vi "RT Main R4.vi"() -> ()   [LabVIEW 2018]
uses:
  Type Defs/Measurement States.ctl
  Type Defs/Control Mode.ctl
  <vilib>/FPGAPlugInAG/myRIO-1900/niLvFpga_Open_myRIO-1900.vi
  <vilib>/rvi/interface/common/dynamic/niFpgaDynamicAddResources.vi
  Global Variables/RT Loop Stop.vi
  <vilib>/Utility/error.llb/Error Cluster From Error Code.vi
  <vilib>/rvi/errors/niLvFpgaAdjustHostInterfaceError.vi
  <vilib>/RVI Host/nirviSupport.llb/nirviErrorClusterFromErrorCode.vi
  <vilib>/rvi/interface/nirviOpenFPGA/nirviOpenFPGA.xnode
  FPGA Bitfiles/WattBalanceRev1_FPGATarget_FPGAMain_doRdIs9Lwbc.lvbitx
  FPGA/FPGA Main R4 One Loop AB JC KV.vi
  <vilib>/rvi/interface/nirviReadWriteControl/nirviReadWriteControl.xnode
  <vilib>/rvi/interface/nirviMethod/nirviMethod.xnode
  Support Libraries/Message Queue/Message Queue.lvlib
  <vilib>/rvi/interface/nirviMethod/StockFPGA_InlinedMethodWaitForSingleIRQ.vi
  <vilib>/FPGAPlugInAG/Dynamic/niLvFpga_WaitOnIrq_Dynamic.vi
  <vilib>/FPGAPlugInAG/Dynamic/niLvFpga_AcknowledgeIrq_Dynamic.vi
  NiFpgaLv.dll
  <vilib>/rvi/interface/Simulation/niFpgaSimulationCallBeginRW.vi
panel:
  out "back emf":i32[](graph)
  out "cap probe":i32[](graph)
  out "IRQ Timeout":bool
  in  "Measure BL":bool
  out "data out":i32[][](array[numeric])
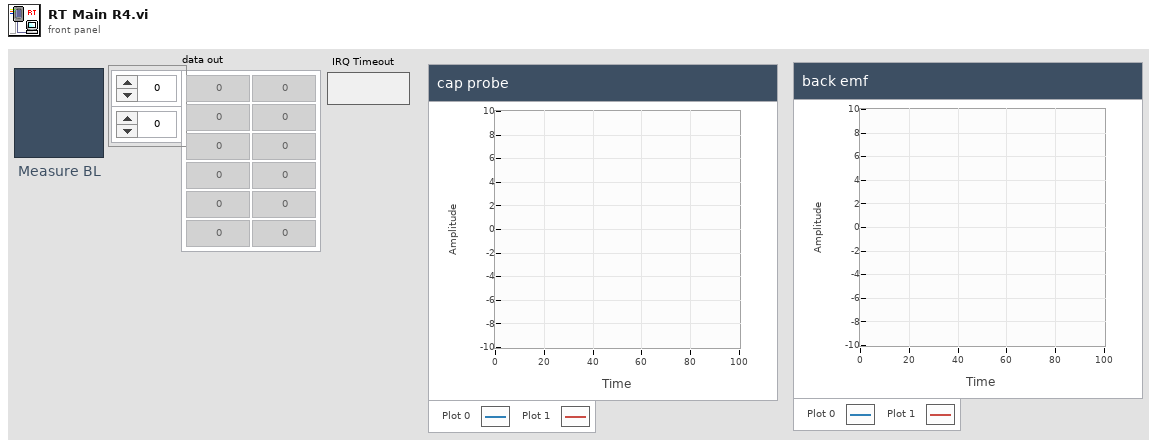
[diagram p1: front panel]
types:
  T1 = typedef "Measurement States.ctl" = enum16{"Idle", "Initialize", "Measure", "Collect Data", "Calculate", "Close"}
  T2 = typedef "Control Mode.ctl" = enum16{"Start Velocity", "Velocity", "End Velocity", "Displacement", "Manual"}
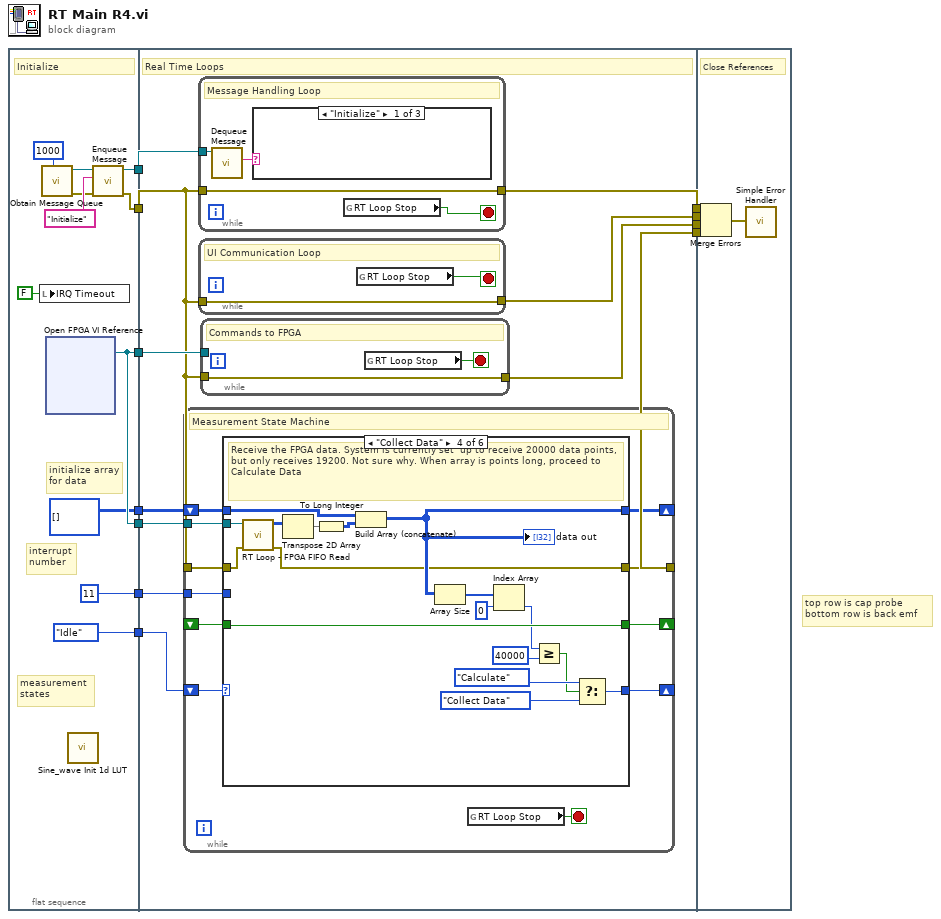
[diagram p0: block diagram]
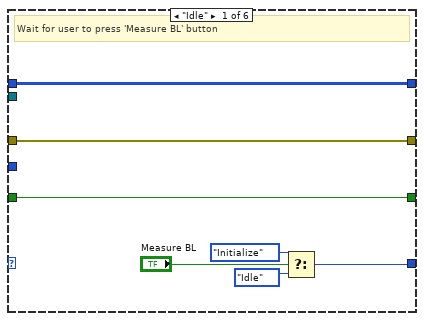
[diagram p4: hidden frame]
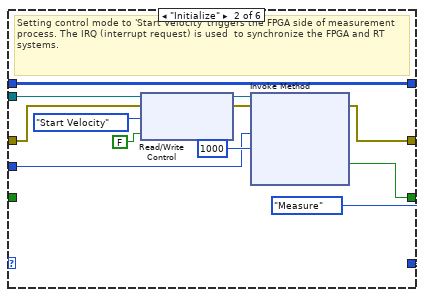
[diagram p5: hidden frame]
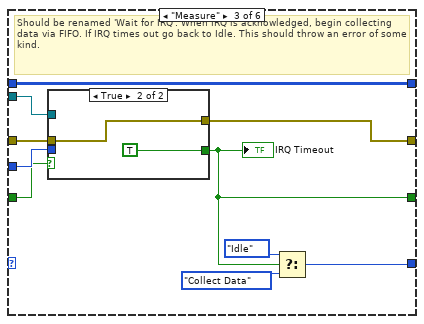
[diagram p6: hidden frame]
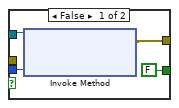
[diagram p7: hidden frame]
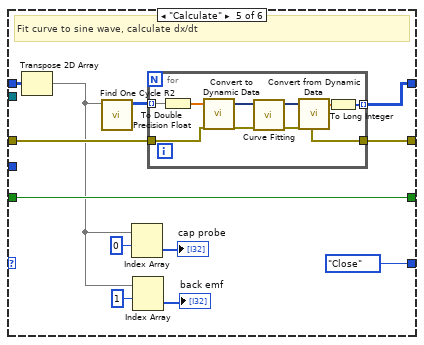
[diagram p8: hidden frame]
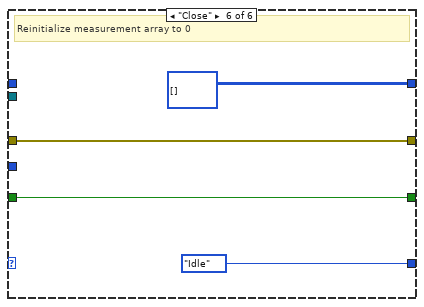
[diagram p9: hidden frame]
diagram:
  # "top row is cap probe\nbottom row is back emf"
  n1 = flat-sequence {
    tunnel: [w16] -> w11
    tunnel: [w15] -> w10
    tunnel: [Measurement_States."Idle" ("Enum")] -> w8
    tunnel: [w18] -> w7
    tunnel: [w15] -> w3
    tunnel: [11 ("IRQ Number(s)")] -> w2
    tunnel: [i32[][] []] -> w1
    tunnel: w11 -> [w25]
    tunnel: w10 -> [w30]
    tunnel: [w33] -> w9
    tunnel: w8 -> [w32]
    tunnel: w7 -> [w31]
    tunnel: [w29] -> w6
    tunnel: [w28] -> w5
    tunnel: [w27] -> w4
    tunnel: w3 -> [w26]
    tunnel: w2 -> [w24]
    tunnel: w1 -> [w23]
    tunnel: w9 -> [w129]
    tunnel: w6 -> [w132]
    tunnel: w5 -> [w131]
    tunnel: w4 -> [w130]
    frame #0 {
      # "measurement\nstates"
      # "interrupt\nnumber"
      # "initialize array\nfor data"
      # "Initialize"
      n2 = local write "IRQ Timeout"(FALSE ("IRQ Timeout")) -> ()
      n3 = call "Obtain Message Queue.vi"("max queue size (-1, unlimited)"=1000) -> ("error out"=w17:errorcluster, "Message Queue"=w20:refnum<queue>)  [unwired: 9 in]
      n4 = xnode "Open FPGA VI Reference"() -> ("FPGA VI Reference Out"=w15:refnum<k20>)  [unwired: 2 in, 1 out]
      n5 = call "Sine_wave Init 1d LUT.vi"() -> ()  [unwired: 11 in, 1 out]
      n6 = call "Enqueue Message.vi"("error in (no error)"=w17, "Message"="Initialize", "Message Queue"=w20) -> ("error out"=w16:errorcluster, "dup Message Queue"=w18:refnum<queue>)  [unwired: 7 in]
    }
    frame #1 {
      # "Real Time Loops"
      n7 = while {
        tunnel: w25 -> [w42]
        tunnel: [w48] -> w33
        shift-right: [w50] -> _
        shift-left: w32 -> [w52]
        tunnel: w26 -> [w49]
        tunnel: w24 -> [w47]
        shift-right: [w46] -> _
        shift-left: _ -> [w45]
        shift-right: [w43] -> _
        shift-left: w23 -> [w44]
        stop <- w51 stop-if-true
        # "Measurement State Machine"
        n8 = case shown="\"Collect Data\"" w52 {
          tunnel: [w57 Measurement_States."Measure" ("Enum") w76 w95 Measurement_States."Close" ("Enum") Measurement_States."Idle" ("Enum")] -> w50
          tunnel: w49 -> [_ w70 w75 w102 _ _]
          tunnel: [w53 w60 w73 w90 w112 w125] -> w48
          tunnel: w47 -> [_ w66 w81 _ _ _]
          tunnel: [w55 w65 w77 w103 w115 w127] -> w46
          tunnel: w45 -> [w55 _ w80 w103 w115 w127]
          tunnel: w44 -> [w54 w63 w74 w93 w107 _]
          tunnel: [w54 w63 w74 w92 w111 u16[][] []] -> w43
          tunnel: w42 -> [w53 w61 w72 w91 w114 w125]
          frame "Idle" {
            # "Wait for user to press 'Measure BL' button"
            n9 = Select(t=Measurement_States."Initialize" ("Enum"), s="Measure BL", f=Measurement_States."Idle" ("Enum")) -> (s? t:f=w57:T1)
          }
          frame "Initialize" {
            # "Setting control mode to 'Start Velocity' triggers the FPGA side of measurement process. The IRQ (interrupt request) is used  to synchronize the FPGA and RT systems."
            n10 = xnode "Read/Write Control"("FPGA VI Reference In"=w70, "error in"=w61, "Control Mode"=Control_Mode."Start Velocity", "FFWD/PID"=FALSE) -> ("FPGA VI Reference Out"=w69:refnum<k20>, "error out"=w68:errorcluster)
            n11 = xnode "Invoke Method"("FPGA VI Reference In"=w69, "error in"=w68, "IRQ Number(s)"=w66, "Timeout (ms)"=1000) -> ("error out"=w60:errorcluster, "Timed Out"=w65:bool)  [unwired: 2 out]
          }
          frame "Measure" {
            # "Should be renamed 'Wait for IRQ'. When IRQ is acknowledged, begin collecting data via FIFO. If IRQ times out go back to Idle. This should throw an error of some kind."
            n12 = case shown="True" w80 {
              tunnel: w75 -> [w85 _]
              tunnel: w81 -> [w84 _]
              tunnel: [FALSE TRUE] -> w77
              tunnel: [w82 w86] -> w73
              tunnel: w72 -> [_ w86]
              frame False {
                n13 = xnode "Invoke Method"("FPGA VI Reference In"=w85, "IRQ Number(s)"=w84) -> ("error out"=w82:errorcluster)  [unwired: 1 in, 1 out]
              }
              frame True {
              }
            }
            "IRQ Timeout" <- w77
            n14 = Select(t=Measurement_States."Idle" ("Enum"), s=w77, f=Measurement_States."Collect Data" ("Enum")) -> (s? t:f=w76:T1)
          }
          frame "Collect Data" {
            # "Receive the FPGA data. System is currently set  up to receive 20000 data points, but only receives 19200. Not sure why. When array is points long, proceed to Calculate Data"
            n15 = call "RT Loop - FPGA FIFO Read.vi"("error in (no error)"=w91, "FPGA VI Reference In"=w102) -> ("error out"=w90:errorcluster, "Data Out"=w104:u16[][])  [unwired: 8 in]
            n16 = Transpose 2D Array(2D array=w104) -> (transposed array=w89:u16[][])
            n17 = To Long Integer(number=w89) -> (32bit integer=w88:i32[][])
            n18 = Build Array (concatenate)(w93, w88) -> (w92:i32[][])
            "data out" <- w92
            n19 = Array Size(array=w92) -> (size(s)=w100:i32[])
            n20 = Index Array(array=w100, index=0) -> (element=w98:i32)
            n21 = Greater Or Equal?(x=w98, y=40000) -> (x >= y?=w94:bool)
            n22 = Select(t=Measurement_States."Calculate" ("Enum"), s=w94, f=Measurement_States."Collect Data" ("Enum")) -> (s? t:f=w95:T1)
          }
          frame "Calculate" {
            # "Fit curve to sine wave, calculate dx/dt"
            n23 = Transpose 2D Array(2D array=w107) -> (transposed array=w105:i32[][])
            n24 = call "Find One Cycle R2.vi"("data in"=w105) -> ("data out"=w113:i32[][])  [unwired: 9 in, 1 out]
            n25 = Index Array(array=w105, index (row)=0) -> (element=→"cap probe":i32[])  [unwired: 1 in]
            n26 = Index Array(array=w105, index (row)=1) -> (element=→"back emf":i32[])  [unwired: 1 in]
            n27 = for {
              tunnel: w114 -> [w123]
              tunnel: w113 -> [w118] mode=indexing
              tunnel: [w122] -> w112
              tunnel: [w119] -> w111 mode=indexing
              n28 = To Double Precision Float(number=w118) -> (double precision float=w117:dbl[])
              n29 = call "Convert to Dynamic Data"("Array"=w117) -> ("Dynamic Data Type"=w124:dynamicdata)  [unwired: 3 in]
              n30 = call "Curve Fitting"("error in (no error)"=w123, "Signals"=w124) -> ("error out"=w122:errorcluster, "best fit"=w121:dynamicdata)  [unwired: 5 in, 3 out]
              n31 = call "Convert from Dynamic Data"("Dynamic Data Type"=w121) -> ("Array"=w120:dbl[])  [unwired: 3 in]
              n32 = To Long Integer(number=w120) -> (32bit integer=w119:i32[])
            }
          }
          frame "Close" {
            # "Reinitialize measurement array to 0"
          }
        }
        n33 = global read "RT Loop Stop.vi" "RT Loop Stop"() -> (w51:bool)
      }
      n34 = while {
        tunnel: w25 -> [w39]
        tunnel: w31 -> [w41]
        tunnel: [w39] -> w29
        stop <- w38 stop-if-true
        # "Message Handling Loop"
        n35 = call "Dequeue Message.vi"("Message Queue"=w41) -> ("Message"=w40:string)  [unwired: 7 in, 3 out]
        n36 = case shown="\"Initialize\"" w40 {
          frame "Initialize" {
          }
          frame Default {
          }
          frame "Exit" {
          }
        }
        n37 = global read "RT Loop Stop.vi" "RT Loop Stop"() -> (w38:bool)
      }
      n38 = while {
        tunnel: [w35] -> w27
        tunnel: w25 -> [w35]
        stop <- w34 stop-if-true
        # "UI Communication Loop"
        n39 = global read "RT Loop Stop.vi" "RT Loop Stop"() -> (w34:bool)
      }
      n40 = while {
        tunnel: w30 -> [_]
        tunnel: w25 -> [w36]
        tunnel: [w36] -> w28
        stop <- w37 stop-if-true
        # "Commands to FPGA"
        n41 = global read "RT Loop Stop.vi" "RT Loop Stop"() -> (w37:bool)
      }
    }
    frame #2 {
      # "Close References"
      n42 = Merge Errors(w132, w130, w131, w129) -> (w133:errorcluster)
      n43 = call <vilib>:"Simple Error Handler.vi"("error in (no error)"=w133) -> ()  [unwired: 4 in, 5 out]
    }
  }
